vi "Logic Gates.vi"() -> ()   [LabVIEW 2024]
panel:
  in  "Boolean 14":bool
  out "Boolean 13":bool
  in  "Numeric 12":dbl
  out "Numeric 11":dbl
  in  "Numeric 10":dbl
  in  "Boolean 12":bool
  out "Boolean 11":bool
  in  "Boolean 10":bool
  in  "Numeric 9":dbl
  out "Numeric 8":dbl
  in  "Numeric 7":dbl
  in  "Boolean 9":bool
  out "Boolean 8":bool
  in  "Boolean 7":bool
  in  "Numeric 6":dbl
  out "Numeric 5":dbl
  in  "Numeric 4":dbl
  in  "Numeric 3":dbl
  out "Numeric 2":dbl
  in  "Numeric":dbl
  in  "Boolean 6":bool
  out "Boolean 5":bool
  in  "Boolean 4":bool
  in  "Boolean 3":bool
  out "Boolean 2":bool
  in  "Boolean":bool
  # "NOT AND\n\n\n\nAND"
  # "OR\n\n\nNOT OR"
  # "NOT"
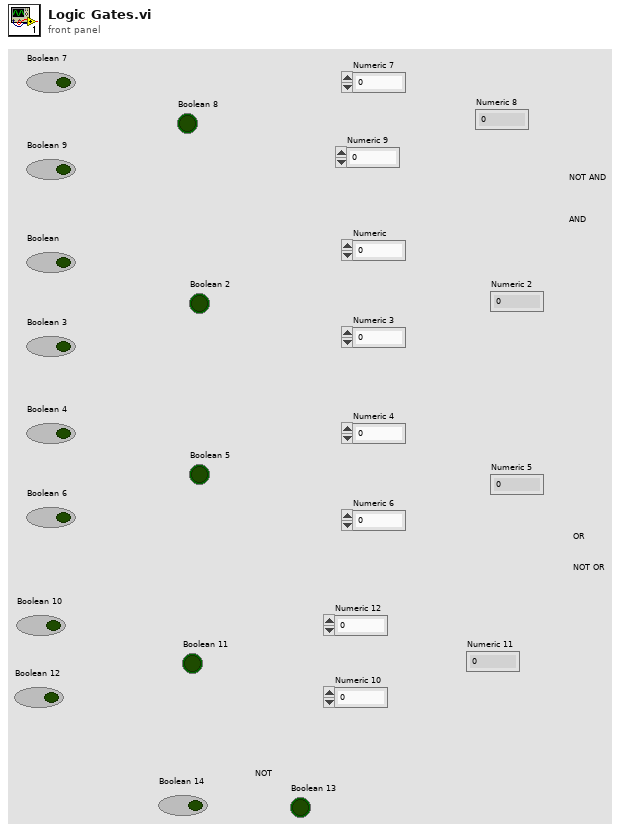
[diagram p1: front panel]
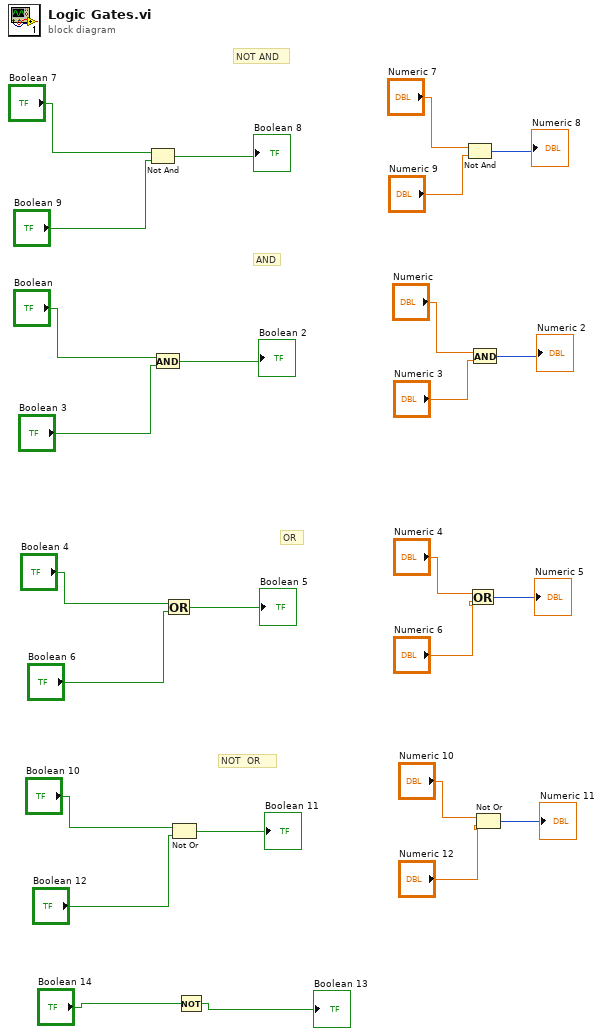
[diagram p0: block diagram]
diagram:
  # "NOT  OR"
  # "NOT AND"
  # "OR"
  # "AND"
  n1 = Not And(1:"Boolean 9", 2:"Boolean 7") -> (0:→"Boolean 8":bool)
  n2 = And(x="Boolean", y="Boolean 3") -> (x .and. y?=→"Boolean 2":bool)
  n3 = Or(x="Boolean 4", y="Boolean 6") -> (x .or. y?=→"Boolean 5":bool)
  n4 = Not Or(1:"Boolean 12", 2:"Boolean 10") -> (0:→"Boolean 11":bool)
  n5 = Not(x="Boolean 14") -> (.not. x?=→"Boolean 13":bool)
  n6 = Not And(1:"Numeric 9", 2:"Numeric 7") -> (0:→"Numeric 8":i32)
  n7 = Or(x="Numeric 4", y="Numeric 6") -> (x .or. y?=→"Numeric 5":i32)
  n8 = And(x="Numeric", y="Numeric 3") -> (x .and. y?=→"Numeric 2":i32)
  n9 = Not Or(1:"Numeric 12", 2:"Numeric 10") -> (0:→"Numeric 11":i32)
